vi "Data Conversion.vi"() -> ()   [LabVIEW 2017]
uses:
  Source/Shared/Typedefs/DSF.Shared.Typedefs.Configuration.Transfer.Channel Block Descriptor.ctl
  Source/Shared/Typedefs/DSF.Shared.Typedefs.Configuration.Transfer.Channel Descriptor.ctl
  Source/Shared/Typedefs/DSF.Shared.Typedefs.Configuration.Transfer.Channel Parameters.ctl
  Source/Shared/Typedefs/DSF.Shared.Typedefs.Data Type.ctl
  Source/Engine/Classes/Buffer/Buffer Converter.lvclass/Buffer Converter.ctl
  Source/Engine/Classes/Buffer/Buffer Converter.lvclass
  Source/Engine/Classes/Buffer/DSF.Engine.Memory.Buffer.lvclass
  Source/DSF.Shared.lvlib
panel:
  in  "channel blocks":T1[](array[typedef]) {"count" format="%d elements"; "First Channel Descriptor"."base address" format="%016x"; "First Channel Descriptor"."Channel Parameters"."offset" format="%d bytes"}
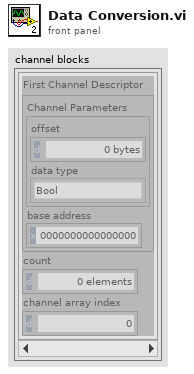
[diagram p1: front panel]
types:
  T1 = typedef "DSF.Shared.lvlib/DSF.Shared.Typedefs.Configuration.Transfer.Channel Block Descriptor.ctl" = cluster{"First Channel Descriptor":T2, "count":u64, "channel array index":u64}
  T2 = typedef "DSF.Shared.lvlib/DSF.Shared.Typedefs.Configuration.Transfer.Channel Descriptor.ctl" = cluster{"Channel Parameters":T3, "base address":u64}
  T3 = typedef "DSF.Shared.lvlib/DSF.Shared.Typedefs.Configuration.Transfer.Channel Parameters.ctl" = cluster{"offset":u64, "data type":T4}
  T4 = typedef "DSF.Shared.lvlib/DSF.Shared.Typedefs.Data Type.ctl" = enum8{"Bool", "SGL", "DBL", "I8", "I16", "I32", "I64", "U8", "U16", "U32", "U64"}
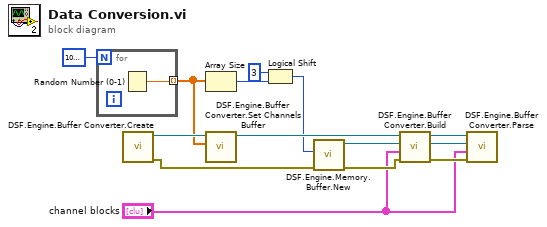
[diagram p0: block diagram]
diagram:
  n1 = for {
    N: 1000000 ("dimension size") -> [_]
    tunnel: [w15] -> w11 mode=indexing
    n2 = Random Number (0-1)() -> (number: 0 to 1=w15:dbl)
  }
  n3 = call "DSF.Engine.Buffer Converter.Create.vi"() -> ("error out"=w8:errorcluster, "Buffer Converter"=w14:refnum<class "Buffer Converter.lvclass">)  [unwired: 10 in]
  n4 = Array Size(array=w11) -> (size(s)=w10:i32)
  n5 = call "DSF.Engine.Buffer Converter.Set Channels Buffer.vi"("channels buffer"=w11, "Buffer Converter in"=w14) -> ("Buffer Converter out"=w13:refnum<class "Buffer Converter.lvclass">)  [unwired: 9 in]
  n6 = Logical Shift(y=i16 3, x=w10) -> (x << y=w6:i32)
  n7 = call "DSF.Engine.Memory.Buffer.New.vi"("error in (no error)"=w8, "size"=w6) -> ("error out"=w7:errorcluster, "Buffer out"=w5:refnum<class "DSF.Engine.Memory.Buffer.lvclass">)  [unwired: 8 in]
  n8 = call "DSF.Engine.Buffer Converter.Build.vi"("error in (no error)"=w7, "channel blocks"="channel blocks", "Buffer in"=w5, "Buffer Converter in"=w13) -> ("error out"=w2:errorcluster, "Buffer out"=w3:refnum<class "DSF.Engine.Memory.Buffer.lvclass">, "Buffer Converter out"=w4:refnum<class "Buffer Converter.lvclass">)  [unwired: 5 in]
  n9 = call "DSF.Engine.Buffer Converter.Parse.vi"("error in (no error)"=w2, "channel blocks"="channel blocks", "Buffer in"=w3, "Buffer Converter in"=w4) -> ()  [unwired: 5 in, 3 out]
